vi "Calculate Data Rate.vi"(0 "total samples":u64, 1 "clear":bool, 5 "last time samples":u64, 11 "last time":dbl) -> (6 "total samples out":u64, 10 "current data rate (bytes/sec)":dbl, 15 "new time":dbl)   [LabVIEW 2016]
doc: "Calculates the data rate.\n\n<B>Input Parameters</B>\n\n<B>total samples</B> specifies the total amount of transferred data.\n\n<B>clear</B> specifies whether to reset the 'Current data rate' to 0.\n\n<B>last time samples</B> specifies the total amount of data transferred the previous time this VI was called.\n\n<B>last time</B> specifies the time at which this VI was previously called.\n\n<B>Output Parameters</B>\n\n<B>total samples out</B> specifies the total amount of transferred data. Use this as 'last time samples' the next time this VI is called.\n\n<B>current data rate (bytes/sec)</B> specifies the calculated data rate.\n\n<B>new time</B> specifies the time at which this VI was called. Use this as 'last time' the next time this VI is called."
uses:
  <vilib>/ptbypt/NI_PtbyPt.lvlib
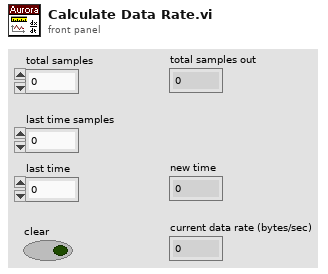
[diagram p1: front panel]
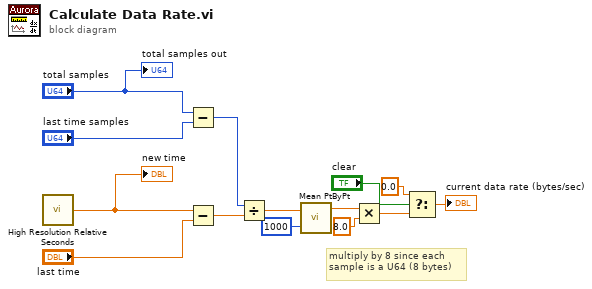
[diagram p0: block diagram]
diagram:
  # "multiply by 8 since each sample is a U64 (8 bytes)"
  n1 = call <vilib>:"High Resolution Relative Seconds.vi"() -> ("relative seconds"=w11:dbl)
  "new time" <- w11
  n2 = Subtract(x="total samples", y="last time samples") -> (x-y=w7:u64)
  n3 = Subtract(x=w11, y="last time") -> (x-y=w13:dbl)
  n4 = Divide(x=w7, y=w13) -> (x/y=w9:dbl)
  n5 = call <vilib>:"Mean PtByPt.vi"("x"=w9, "sample length"=1000) -> ("mean"=w5:dbl)  [unwired: 2 in, 1 out]
  n6 = Multiply(x=w5, y=8.0) -> (x*y=w3:dbl)
  n7 = Select(t=0.0, s="clear", f=w3) -> (s? t:f=→"current data rate (bytes/sec)":dbl)
  "total samples out" <- "total samples"
